vi "5004 VI Name Not Found.vi"(8 "error in (no error)":errorcluster, 11 "VI Name":string) -> (0 "error out":errorcluster)   [LabVIEW 2020, in "MacroAssert.lvlib" / "Custom Errors.lvlib"]
uses:
  Custom Errors.lvlib
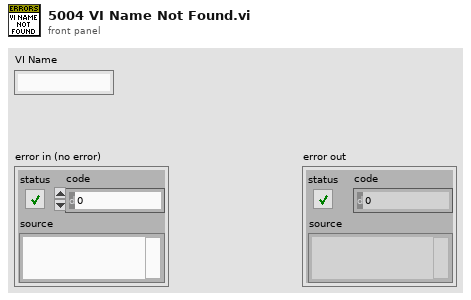
[diagram p1: front panel]
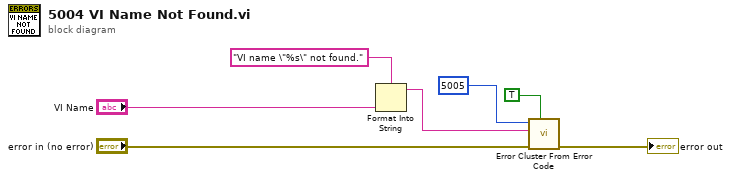
[diagram p0: block diagram]
diagram:
  n1 = Format Into String(format string="VI name \"%s\" not found.", "VI Name") -> (resulting string=w2:string)  [unwired: 2 in, 1 out]
  n2 = call <vilib>:"Error Cluster From Error Code.vi"("show call chain? (False)"=TRUE, "error in (no error)"="error in (no error)", "error message (\"\")"=w2, "error code (0)"=5005) -> ("error out"=→"error out":errorcluster)  [unwired: 5 in]
